vi "write_json.vi"(8 "error in (no error)":errorcluster, 10 "json":string, 11 "json.provider in":refnum<class "json.provider.lvclass">) -> (0 "error out":errorcluster, 3 "json.provider out":refnum<class "json.provider.lvclass">)   [LabVIEW 2021, in "json.provider.lvclass"]
uses:
  json.provider.lvclass
  json.provider.lvclass/json.provider.ctl
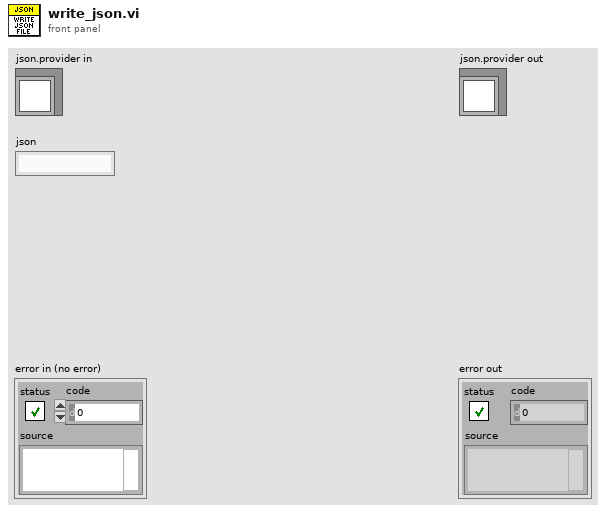
[diagram p1: front panel]
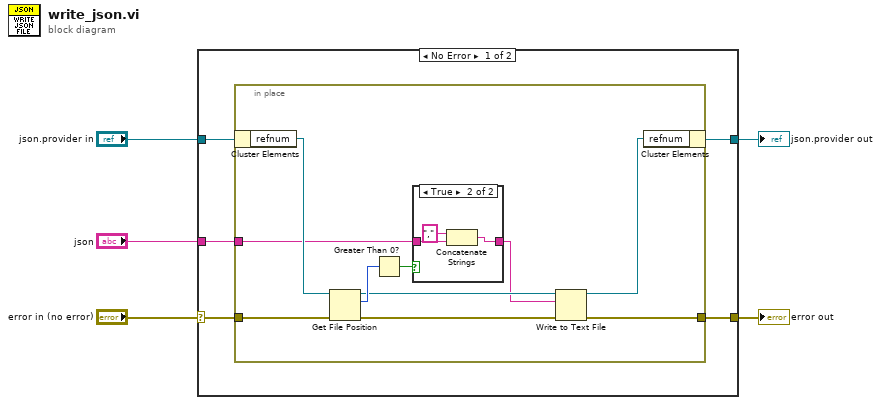
[diagram p0: block diagram]
diagram:
  n1 = case shown="No Error" "error in (no error)" {
    selector: "error in (no error)" -> [w8 w26]
    tunnel: [w7 w26] -> w4
    tunnel: [w9 w25] -> w2
    tunnel: "json.provider in" -> [w10 w25]
    tunnel: "json" -> [w6 _]
    frame No Error {
      n2 = in-place {
        in-place-border: w8 -> [w19]
        in-place-border: [w20] -> w7
        in-place-border: w6 -> [w13]
        n3 = in-place-cluster #1(w10) -> ("refnum"=w18:refnum<file>)
        n4 = Get File Position(4:w19, 7:w18) -> (0:w16:errorcluster, 2:w17:i64, 3:w15:refnum<file>)
        n5 = Greater Than 0?(x=w17) -> (x > 0?=w14:bool)
        n6 = case shown="True" w14 {
          tunnel: w13 -> [w21 w24]
          tunnel: [w21 w23] -> w12
          frame False {
          }
          frame True {
            n7 = Concatenate Strings("," ("string"), w24) -> (w23:string)
          }
        }
        n8 = Write to Text File(file (use dialog)=w15, text=w12, error in=w16) -> (refnum out=w11:refnum<file>, error out=w20:errorcluster)  [unwired: 1 in, 1 out]
        n9 = in-place-cluster #1("refnum"=w11) -> (w9:refnum<class "json.provider.lvclass">)
      }
    }
    frame Error {
    }
  }
  "error out" <- w4
  "json.provider out" <- w2
